vi "PCO_OpenCamera.vi"(8 "error in (no error)":errorcluster {"code" format="%x"}) -> (0 "error out":errorcluster {"code" format="%x"}, 2 "ErrorMessage":i32 format="%x", 3 "ph out":u64)   [LabVIEW 2019, in "SDK.lvlib" / "CameraAccess.lvlib"]
doc: "<b>Description:</b>\nThis function is used to get a connection to a camera. A unique handle is returned, which must be used for all other function calls. This function scans through all available interfaces and tries to connect to the next available camera. If more than one camera is connected to the computer this function must be called a second time to get the handle for the next camera. If a distinct camera should be accessed PCO_OpenCameraEx has to be used.\nBecause this function is using a scan process wCamNum parameter is not used.\n\n<b>Supported camera type:</b>\nAll cameras\n\n<b>Descriptor dependency:</b>\nNone"
uses:
  CameraAccess.lvlib
panel:
  in  "wCamNum":u16
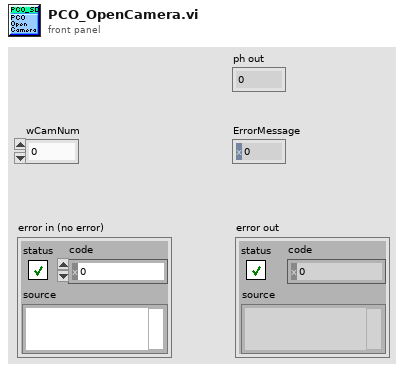
[diagram p1: front panel]
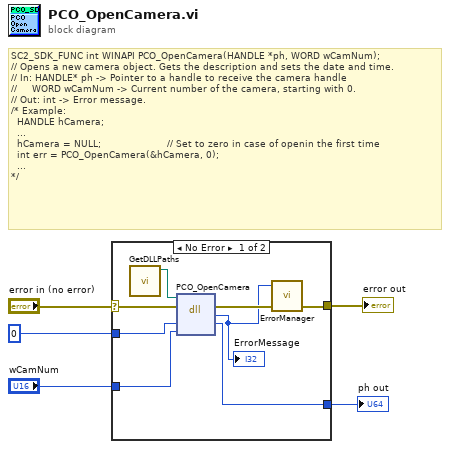
[diagram p0: block diagram]
diagram:
  # "SC2_SDK_FUNC int WINAPI PCO_OpenCamera(HANDLE *ph, WORD wCamNum);\n// Opens a new camera object. Gets the description and sets the date and time.\n// In: HANDLE* ph -> Pointer to a handle to receive the camera handle\n//     WORD wCamNum -> Current number of the camera, starting with 0.\n// Out: int -> Error message.\n/* Example:\n  HANDLE hCamera;\n  ...\n  hCamera = NULL;                      // Set to zero in case of openin the first time\n  int err = PCO_OpenCamera(&hCamera, 0);\n  ...\n*/"
  n1 = case shown="No Error" "error in (no error)" {
    selector: "error in (no error)" -> [w13 w15]
    tunnel: [w11 w15] -> w5
    tunnel: u64 0 -> [w9 w14]
    tunnel: [w8 w14] -> w3
    tunnel: "wCamNum" -> [w7 _]
    frame No Error {
      n2 = call "GetDLLPaths.vi"() -> ("SC2_Cam_Path"=w6:path)  [unwired: 9 in, 2 out]
      n3 = dll-call lib="?" fn="PCO_OpenCamera"(path in=w6, error in=w13, "ph"=w9, "wCamNum"=w7) -> (error out=w12:errorcluster, "return type"=w10:i32, "ph"=w8:u64)  [unwired: 2 in, 1 out]
      "ErrorMessage" <- w10
      n4 = call "ErrorManager.vi"("error in (no error)"=w12, "error code"=w10) -> ("error out"=w11:errorcluster)  [unwired: 3 in]
    }
    frame Error {
    }
  }
  "error out" <- w5
  "ph out" <- w3
